vi "LS Das Bank2 Error Index.vi"(0 "RowCountSlow":i32, 5 "SlowRecordIndexes":i32[](array[numeric]), 7 "Bank2SlowRecord":bool, 9 "RowCountStandard":i32, 11 "ErrorIndex":i32) -> (4 "Bank2ErrorIndex":string)   [LabVIEW 2019]
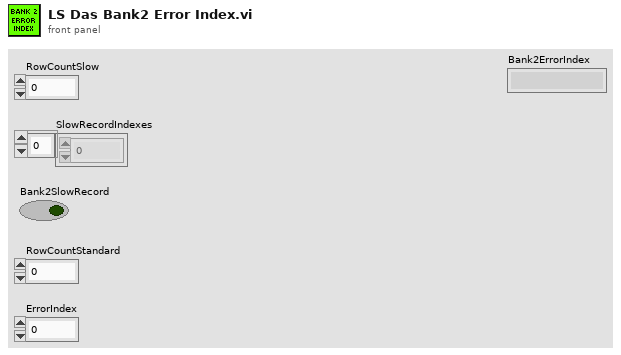
[diagram p1: front panel]
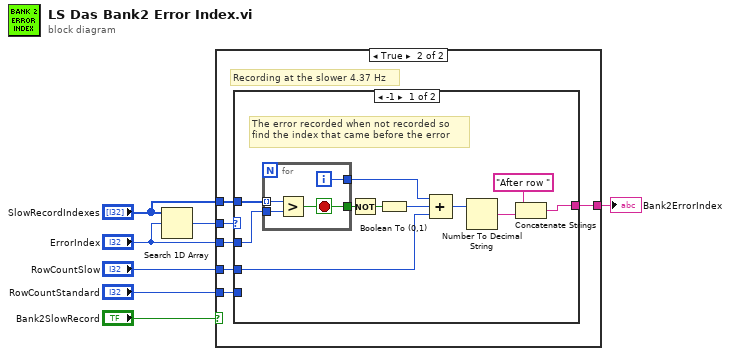
[diagram p0: block diagram]
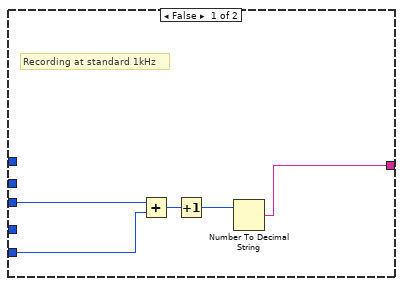
[diagram p2: hidden frame]
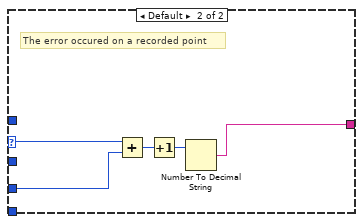
[diagram p3: hidden frame]
diagram:
  n1 = Search 1D Array(1D array="SlowRecordIndexes", element="ErrorIndex") -> (index of element=w7:i32)  [unwired: 1 in]
  n2 = case shown="True" "Bank2SlowRecord" {
    tunnel: w7 -> [_ w18]
    tunnel: "RowCountSlow" -> [_ w17]
    tunnel: "SlowRecordIndexes" -> [_ w16]
    tunnel: "ErrorIndex" -> [w11 w15]
    tunnel: "RowCountStandard" -> [w12 w13]
    tunnel: [w10 w14] -> w1
    frame False {
      # "Recording at standard 1kHz"
      n3 = Add(x=w11, y=w12) -> (x+y=w9:i32)
      n4 = Increment(x=w9) -> (x+1=w8:i32)
      n5 = Number To Decimal String(number=w8) -> (decimal integer string=w10:string)  [unwired: 1 in]
    }
    frame True {
      # "Recording at the slower 4.37 Hz"
      n6 = case shown="-1" w18 {
        selector: w18 -> [_ w38]
        tunnel: w17 -> [w19 w37]
        tunnel: w16 -> [w29 _]
        tunnel: w15 -> [w28 _]
        tunnel: [w23 w34] -> w14
        tunnel: w13 -> [_ _]
        frame -1 {
          # "The error recorded when not recorded so\nfind the index that came before the error"
          n7 = for {
            tunnel: w29 -> [w33] mode=indexing
            tunnel: w28 -> [w32]
            tunnel: [w31] -> w22
            tunnel: [w30] -> w27
            i -> [w31]
            stop <- w30 stop-if-true
            n8 = Greater?(x=w33, y=w32) -> (0:w30:bool)
          }
          n9 = Not(x=w27) -> (.not. x?=w26:bool)
          n10 = Boolean To (0,1)(Boolean=w26) -> (0, 1=w21:i16)
          n11 = Compound Arithmetic op=ADD(w22, w21, w19) -> (w20:i32)
          n12 = Number To Decimal String(number=w20) -> (decimal integer string=w24:string)  [unwired: 1 in]
          n13 = Concatenate Strings("After row ", w24) -> (w23:string)
        }
        frame Default {
          # "The error occured on a recorded point"
          n14 = Add(x=w38, y=w37) -> (x+y=w36:i32)
          n15 = Increment(x=w36) -> (x+1=w35:i32)
          n16 = Number To Decimal String(number=w35) -> (decimal integer string=w34:string)  [unwired: 1 in]
        }
      }
    }
  }
  "Bank2ErrorIndex" <- w1
